vi "Matrix_AssignBlock.vi"(8 "StartColumn":i32, 9 "StartRow":i32, 10 "Other Matrix":T1, 11 "input matrix":T1) -> (3 "output matrix":T1)   [LabVIEW 2019, in "Trajectory_Library.lvlib"]
doc: "Creates a new LINEAR SYSTEM data cluster with the specified values. \n\n\nInputs: \n - XXX -- XXX.\n\nOutputs:\n - XXX -- XXX."
uses:
  Trajectory_Library.lvlib
  <vilib>/Analysis/Matrix/Datatypes/RealMatrix.ctl
  <vilib>/Analysis/Matrix/NI_Matrix.lvlib
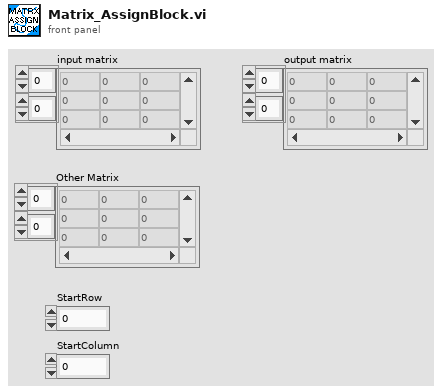
[diagram p1: front panel]
types:
  T1 = typedef "NI_Matrix.lvlib/RealMatrix.ctl" = dbl[][]
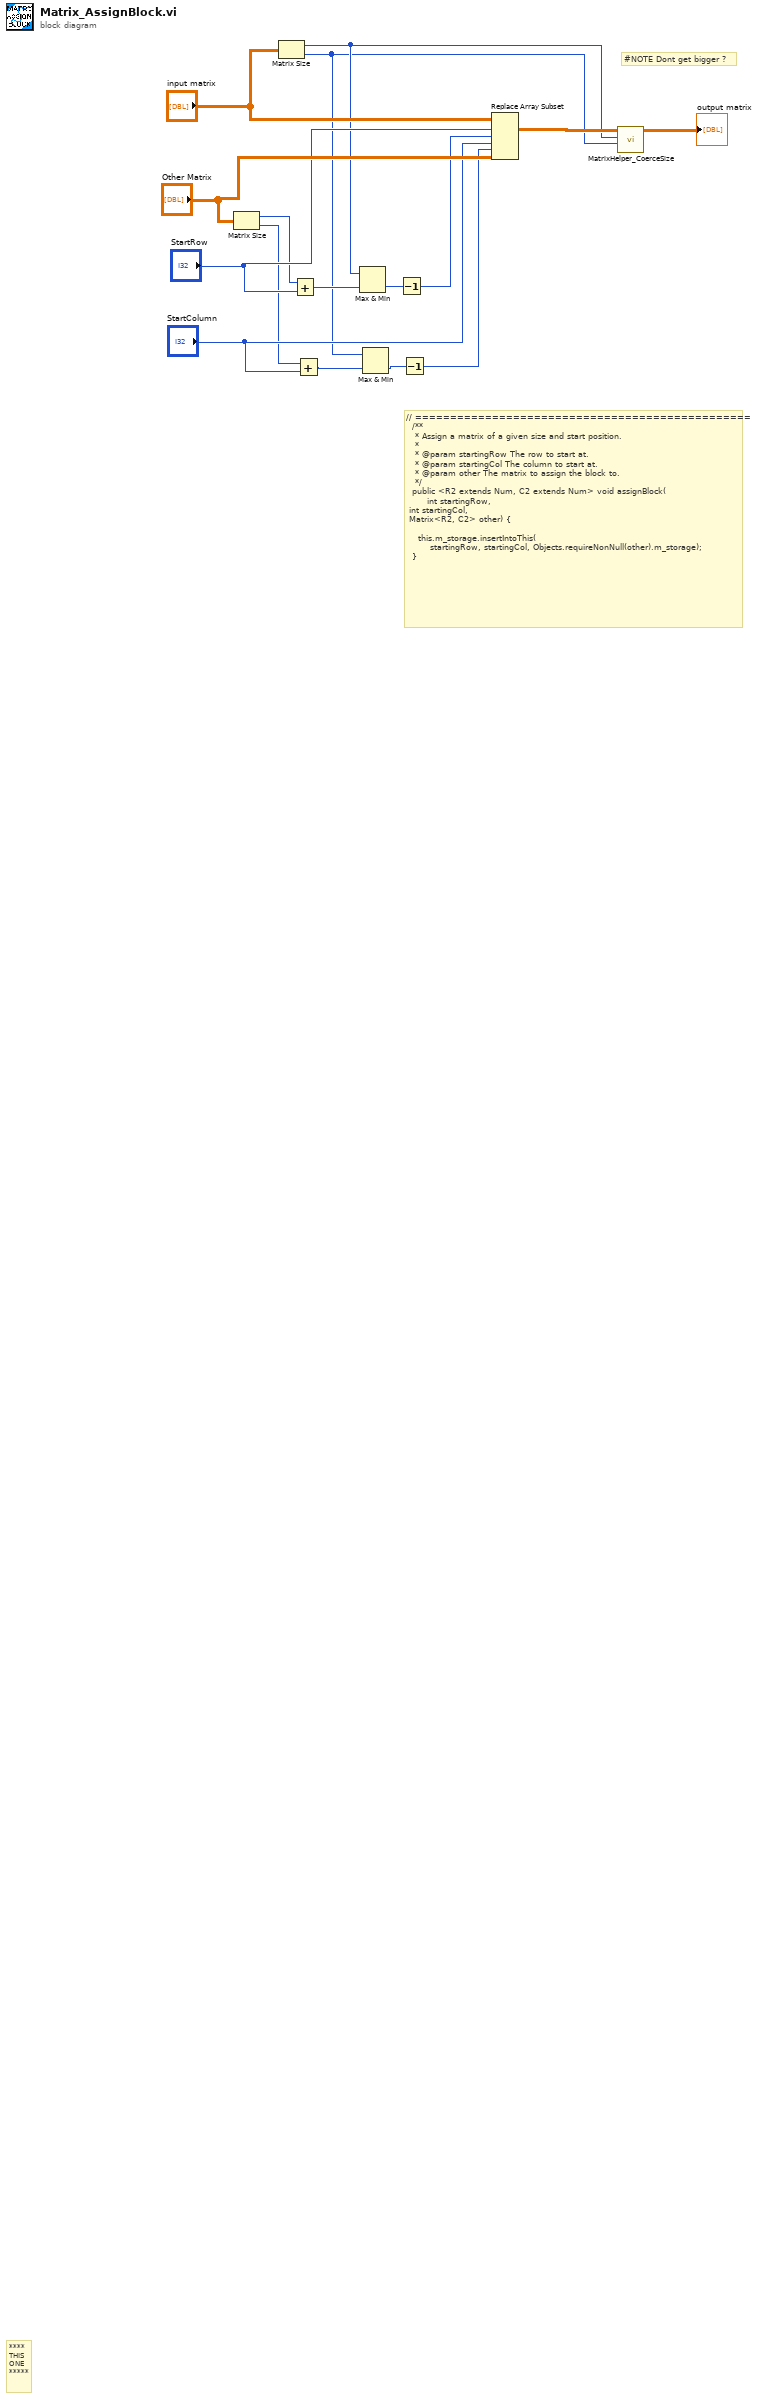
[diagram p0: block diagram]
diagram:
  # "#NOTE Dont get bigger ?"
  # "// ================================================\n  /**\n   * Assign a matrix of a given size and start position.\n   *\n   * @param startingRow The row to start at.\n   * @param startingCol The column to start at.\n   * @param other The matrix to assign the block to.\n   */\n  public <R2 extends Num, C2 extends Num> void assignBlock(\n      \tint startingRow, \n\tint startingCol, \n\tMatrix<R2, C2> other) {\n\n    this.m_storage.insertIntoThis(\n        startingRow, startingCol, Objects.requireNonNull(other).m_storage);\n  }"
  # "****\nTHIS\nONE\n*****"
  n1 = Matrix Size(0:"Other Matrix") -> (1:w12:i32, 2:w10:i32)
  n2 = Matrix Size(0:"input matrix") -> (1:w4:i32, 2:w1:i32)
  n3 = Add(x=w12, y="StartRow") -> (x+y=w5:i32)
  n4 = Add(x=w10, y="StartColumn") -> (x+y=w2:i32)
  n5 = Max & Min(x=w4, y=w5) -> (min(x,y)=w6:i32)  [unwired: 1 out]
  n6 = Max & Min(x=w1, y=w2) -> (min(x,y)=w3:i32)  [unwired: 1 out]
  n7 = Decrement(x=w6) -> (x-1=w9:i32)
  n8 = Decrement(x=w3) -> (x-1=w8:i32)
  n9 = Replace Array Subset(array="input matrix", new element="Other Matrix", index (dim 0)="StartRow", index (dim 1)=w9, index (dim 2)="StartColumn", index (dim 3)=w8) -> (w7:T1)
  n10 = call "MatrixHelper_CoerceSize.vi"("Columns"=w1, "Rows"=w4, "input matrix"=w7) -> ("output matrix"=→"output matrix":T1)  [unwired: 8 in]
